vi "Next Value (SGL).vi"(6 "default timestamp":timestamp, 8 "error in (no error)":errorcluster, 9 "timeout":dbl[unit]=1.0, 10 "default value":sgl, 11 "Subscription in":refnum<class "Subscription.lvclass">) -> (0 "error out":errorcluster, 1 "timed out?":bool, 2 "value":sgl, 3 "Subscription out":refnum<class "Subscription.lvclass">, 4 "timestamp":timestamp, 5 "PV name":string)   [LabVIEW 2020, in "PV Access.lvlib" / "PVA Client.lvlib" / "Subscription.lvclass"]
uses:
  Subscription.lvclass
  PV Data/PV Data/PV Data.lvclass
  53427cec-2bea-4028-8de6-3d4e850a6ab9.vi
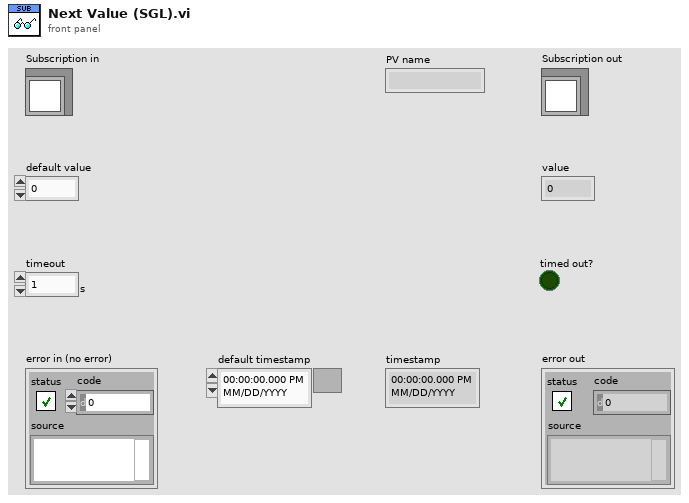
[diagram p1: front panel]
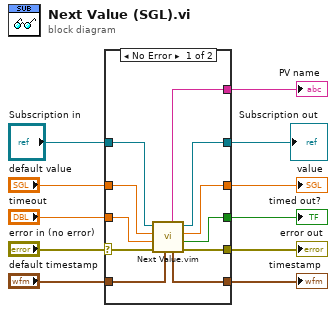
[diagram p0: block diagram]
diagram:
  n1 = case shown="No Error" "error in (no error)" {
    selector: "error in (no error)" -> [w20 w26]
    tunnel: [w19 w26] -> w10
    tunnel: [w21 w25] -> w8
    tunnel: "Subscription in" -> [w22 w25]
    tunnel: "timeout" -> [w18 _]
    tunnel: "default value" -> [w17 w24]
    tunnel: [w16 w24] -> w5
    tunnel: [w15 _] -> w4
    tunnel: [w14 _] -> w3
    tunnel: [w13 w23] -> w2
    tunnel: "default timestamp" -> [w12 w23]
    frame No Error {
      n2 = call "Next Value.vim"("default timestamp"=w12, "error in"=w20, "timeout"=w18, "default value"=w17, "Subscription in"=w22) -> ("error out"=w19:errorcluster, "timed out?"=w15:bool, "value"=w16:sgl, "Subscription out"=w21:refnum<class "Subscription.lvclass">, "timestamp"=w13:timestamp, "PV name"=w14:string)  [unwired: 1 in]
    }
    frame Error {
    }
  }
  "error out" <- w10
  "Subscription out" <- w8
  "value" <- w5
  "timed out?" <- w4
  "PV name" <- w3
  "timestamp" <- w2
